vi "array -- bilinear regression 2D.vi"(7 "action":T5, 10 "fit  IN":dbl[](array[numeric])=[1.9, 2.6, 3.3, 1.0, 2.7, 3.9], 11 "xyz IN":cluster{"x":dbl[], "y":dbl[], "z":dbl[]}={"x"=[0.0, 0.0, 0.0, -1.0, -1.0, -1.0, 1.0, 1.0, 1.0], "y"=[-1.0, 0.0, 1.0, -1.0, 0.0, 1.0, -1.0, 0.0, 1.0], "z"=[1.0, 0.0, 1.0, 4.0, 1.0, 0.0, 0.0, 1.0, 4.0]}) -> (0 "output cluster":T3, 1 "fit map out":map{T4, dbl}(c390)={enum."1"=0.0, enum."x"=0.0, enum."y"=0.0, enum."xx"=1.0, enum."xy"=1.0, enum."yy"=1.0}, 2 "fit OUT":dbl[](array[numeric])=[1.0, 1.0, 1.0, 0.0, 0.0, 0.0], 3 "xyz OUT":cluster{"x":dbl[], "y":dbl[], "z":dbl[]}={"x"=[0.0, 0.0, 0.0, -1.0, -1.0, -1.0, 1.0, 1.0, 1.0], "y"=[-1.0, 0.0, 1.0, -1.0, 0.0, 1.0, -1.0, 0.0, 1.0], "z"=[1.0, 0.0, 1.0, 4.0, 1.0, 0.0, 0.0, 1.0, 4.0]})   [LabVIEW 2020]
uses:
  array -- fit control .ctl
  array -- bilinear regression 2D.ctl
  <vilib>/Analysis/Matrix/Datatypes/RealMatrix.ctl
  <vilib>/Analysis/Matrix/Datatypes/ComplexMatrix.ctl
  <vilib>/Analysis/7linalg.llb/Eigenvalue and Vectors Output Option.ctl
  <vilib>/Analysis/baseanly.llb/Matrix Type of Inverse Matrix.ctl
  <vilib>/Analysis/baseanly.llb/Real A x B.vi
  <vilib>/Analysis/Matrix/Numeric/Conversions/Array To Matrix - RA2.vi
  <vilib>/Analysis/baseanly.llb/Real Inverse Matrix.vi
  <vilib>/Analysis/Matrix/Numeric/Conversions/Matrix To Array - RM.vi
  <vilib>/Analysis/7linalg.llb/Real Eigenvalues and Vectors.vi
  <vilib>/Analysis/Matrix/Numeric/Conversions/Matrix To Array - CM.vi
  <vilib>/Analysis/NI_AALBase.lvlib
  <vilib>/Analysis/Matrix/NI_Matrix.lvlib
  <vilib>/Analysis/NI_AALPro.lvlib
panel:
  out "y OUT":dbl[](array[numeric])=[-1.0, 0.0, 1.0, -1.0, 0.0, 1.0, -1.0, 0.0, 1.0]
  out "y":dbl[](array[numeric])=[-1.0, 0.0, 1.0, -1.0, 0.0, 1.0, -1.0, 0.0, 1.0]
  out "x OUT":dbl[](array[numeric])=[0.0, 0.0, 0.0, -1.0, -1.0, -1.0, 1.0, 1.0, 1.0]
  out "z OUT":dbl[](array[numeric])=[1.0, 0.0, 1.0, 4.0, 1.0, 0.0, 0.0, 1.0, 4.0]
  out "z":dbl[](array[numeric])=[1.0, 0.0, 1.0, 4.0, 1.0, 0.0, 0.0, 1.0, 4.0]
  out "x":dbl[](array[numeric])=[0.0, 0.0, 0.0, -1.0, -1.0, -1.0, 1.0, 1.0, 1.0]
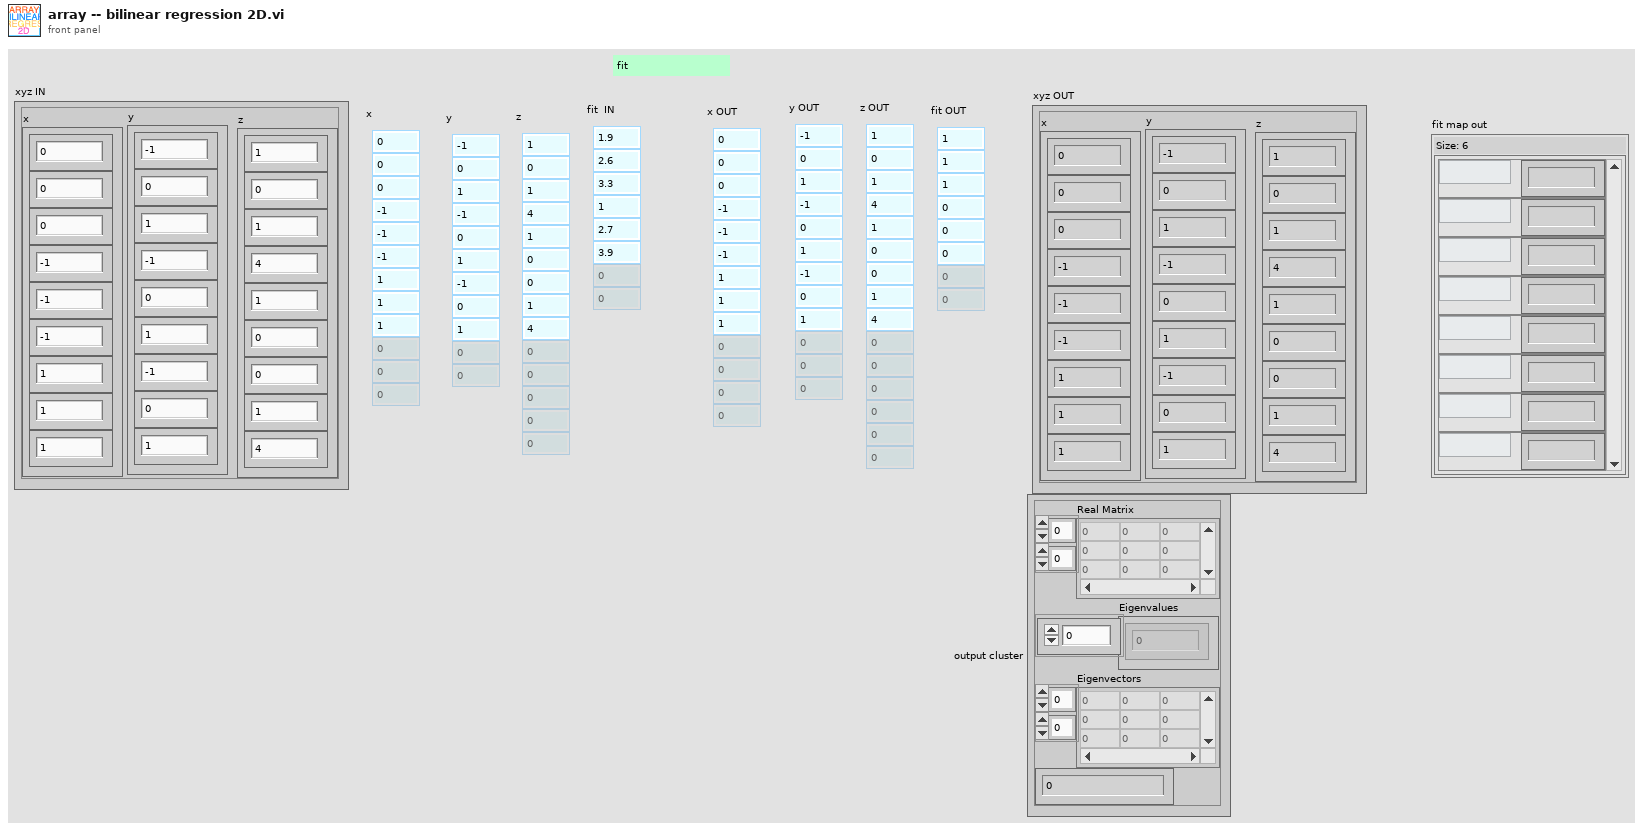
[diagram p1: front panel]
types:
  T1 = typedef "NI_Matrix.lvlib/RealMatrix.ctl" = dbl[][]
  T2 = typedef "NI_Matrix.lvlib/ComplexMatrix.ctl" = cdb[][]
  T3 = cluster{"Real Matrix":T1, "Eigenvalues":cdb[], "Eigenvectors":T2, "Numeric":cdb}
  T4 = typedef "array -- bilinear regression 2D.ctl" = enum16{"1", "x", "y", "xx", "xy", "yy", "xxy", "xyy", "yyy", "xxx", "xxyy", "xyyy", "xxxy", "yyyy", "xxxx", "xxz", "xyz", "yyz", "xz", "yz", "z"}
  T5 = typedef "array -- fit control .ctl" = enum16{"fit", "calc", "check", "init"}
  T6 = typedef "NI_AALPro.lvlib/Eigenvalue and Vectors Output Option.ctl" = i32
  T7 = typedef "NI_AALBase.lvlib/Matrix Type of Inverse Matrix.ctl" = enum32{"General", "Positive Definite", "Lower Triangular", "Upper Triangular"}
  T8 = cluster{"Real Matrix":T1, "Eigenvalues":cdb[], "Eigenvectors":T2, dbl}
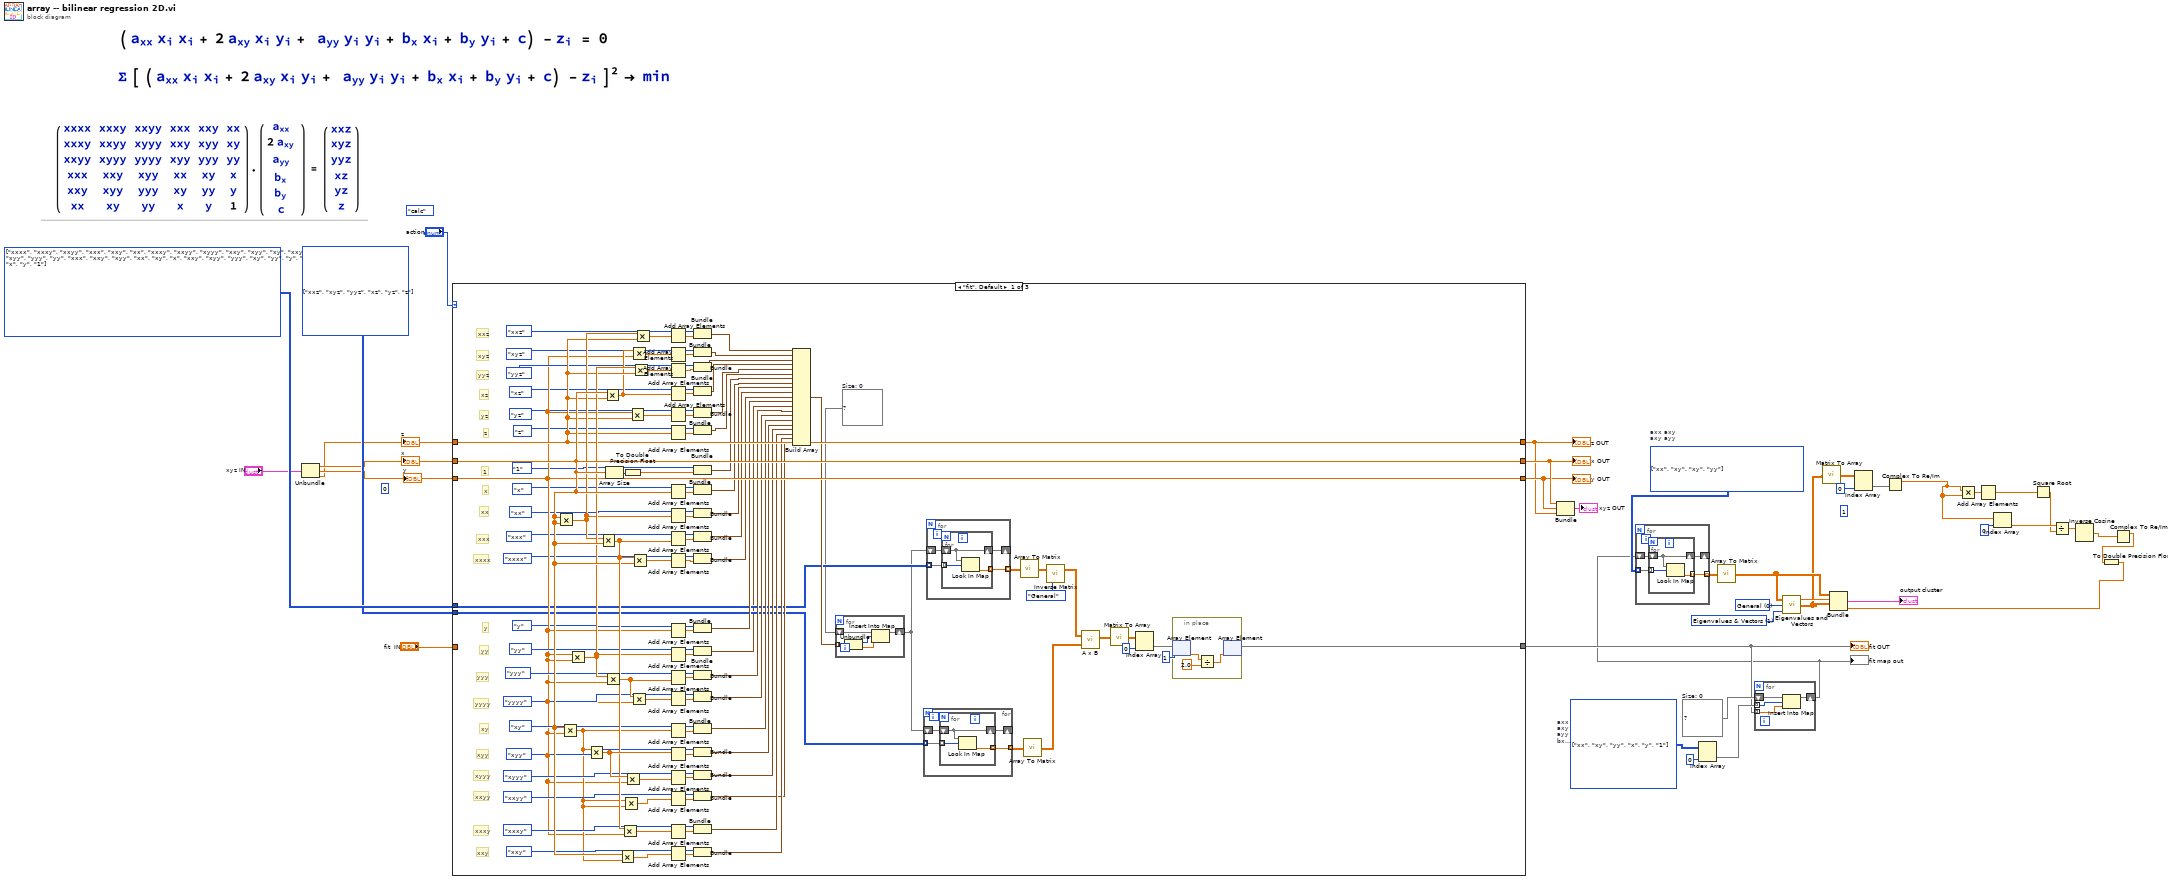
[diagram p0: block diagram]
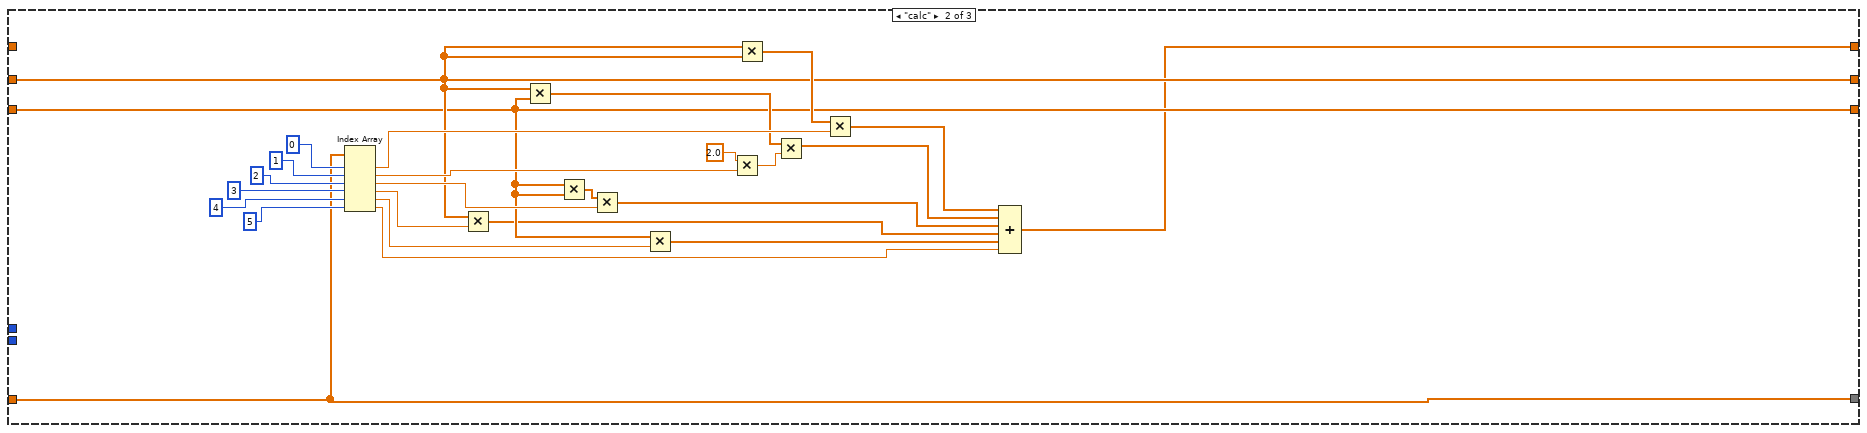
[diagram p2: hidden frame]
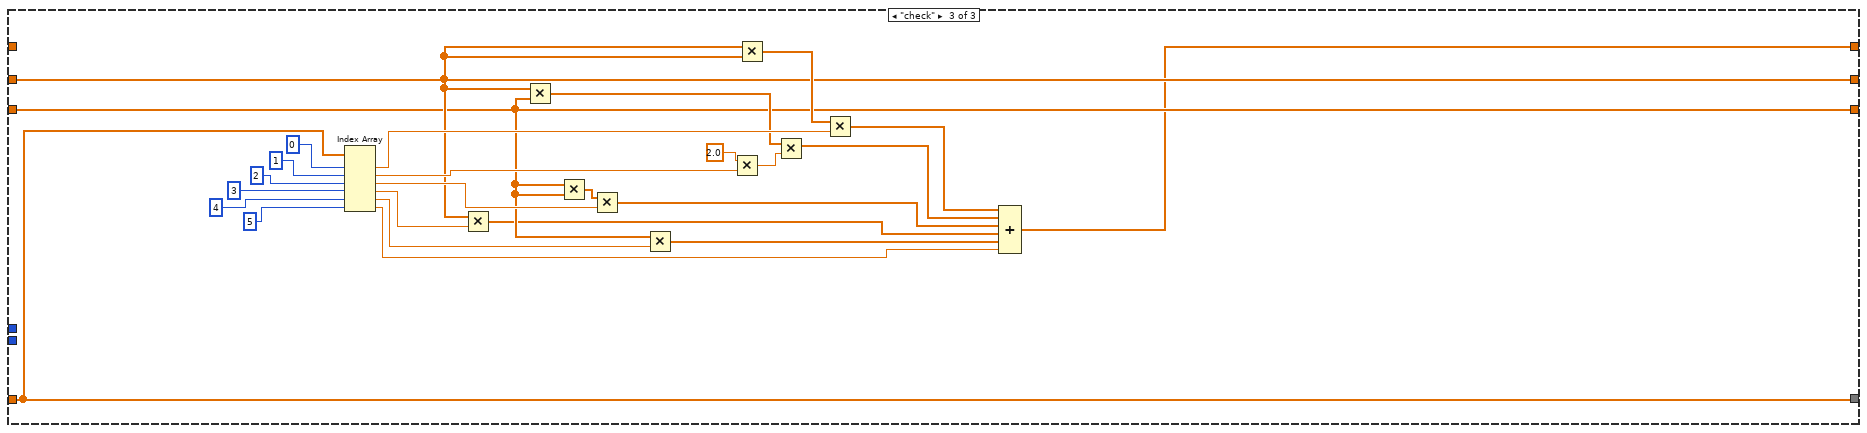
[diagram p3: hidden frame]
diagram:
  (unwired) 1 ("length")
  w18 = map{T4, dbl} {}  # Size: 0
  w20 = T4[][] [[enum."xx"], [enum."xy"], [enum."yy"], [enum."x"], [enum."y"], [enum."1"]] items=["1", "x", "y", "xx", "xy", "yy", "xxy", "xyy", "yyy", "xxx", "xxyy", "xyyy", "xxxy", "yyyy", "xxxx", "xxz", "xyz", "yyz", "xz", "yz", "z"]  # axx axy ayy bx by c
  w24 = T6 1 items=["Eigenvalues", "Eigenvalues & Vectors"] ("output option")
  w23 = 0 items=["General", "Symmetric"] ("matrix type")
  w22 = T4[][] [[enum."xx", enum."xy"], [enum."xy", enum."yy"]] items=["1", "x", "y", "xx", "xy", "yy", "xxy", "xyy", "yyy", "xxx", "xxyy", "xyyy", "xxxy", "yyyy", "xxxx", "xxz", "xyz", "yyz", "xz", "yz", "z"]  # axx axy axy ayy
  (unwired) array_--_fit_control_."calc" ("action")
  w36 = T4[][] [[enum."xxz"], [enum."xyz"], [enum."yyz"], [enum."xz"], [enum."yz"], [enum."z"]] items=["1", "x", "y", "xx", "xy", "yy", "xxy", "xyy", "yyy", "xxx", "xxyy", "xyyy", "xxxy", "yyyy", "xxxx", "xxz", "xyz", "yyz", "xz", "yz", "z"]
  w37 = T4[][] [[enum."xxxx", enum."xxxy", enum."xxyy", enum."xxx", enum."xxy", enum."xx"], [enum."xxxy", enum."xxyy", enum."xyyy", enum."xxy", enum."xyy", enum."xy"], [enum."xxyy", enum."xyyy", enum."yyyy", enum."xyy", enum."yyy", enum."yy"], [enum."xxx", enum."xxy", enum."xyy", enum."xx", enum."xy", enum."x"], [enum."xxy", enum."xyy", enum."yyy", enum."xy", enum."yy", enum."y"], [enum."xx", enum."xy", enum."yy", enum."x", enum."y", enum."1"]] items=["1", "x", "y", "xx", "xy", "yy", "xxy", "xyy", "yyy", "xxx", "xxyy", "xyyy", "xxxy", "yyyy", "xxxx", "xxz", "xyz", "yyz", "xz", "yz", "z"]
  (unwired) 0
  n1 = Unbundle("xyz IN") -> ("x"=w31:dbl[], "y"=w30:dbl[], "z"=w29:dbl[])
  "x" <- w31
  "z" <- w29
  "y" <- w30
  n2 = case shown="\"fit\", Default" "action" {
    tunnel: w29 -> [w122 _ _]
    tunnel: w31 -> [w125 w174 w200]
    tunnel: [w41 w163 w189] -> w17
    tunnel: [w122 w164 w190] -> w33
    tunnel: [w125 w174 w200] -> w35
    tunnel: "fit  IN" -> [_ w163 w189]
    tunnel: w30 -> [w94 w171 w197]
    tunnel: [w94 w171 w197] -> w34
    tunnel: w37 -> [w52 _ _]
    tunnel: w36 -> [w51 _ _]
    frame "fit", Default {
      w42 = map{T4, dbl} {}  # Size: 0
      # "z"
      # "xxz"
      # "yz"
      # "xz"
      # "yyz"
      # "xyz"
      # "xxy"
      # "xxxy"
      # "xxyy"
      # "xyyy"
      # "xyy"
      # "xy"
      # "yyyy"
      # "yyy"
      # "yy"
      # "y"
      # "1"
      # "xxxx"
      # "xxx"
      # "xx"
      # "x"
      n3 = Multiply(x=w125, y=w125) -> (x*y=w123:dbl[])
      n4 = Multiply(x=w125, y=w94) -> (x*y=w102:dbl[])
      n5 = Multiply(x=w94, y=w94) -> (x*y=w124:dbl[])
      n6 = Multiply(x=w102, y=w94) -> (x*y=w131:dbl[])
      n7 = Multiply(x=w123, y=w125) -> (x*y=w128:dbl[])
      n8 = Multiply(x=w125, y=w122) -> (x*y=w120:dbl[])
      n9 = Multiply(x=w124, y=w94) -> (x*y=w135:dbl[])
      n10 = Array Size(array=w125) -> (size(s)=w83:i32)
      n11 = Multiply(x=w125, y=w102) -> (x*y=w129:dbl[])
      n12 = Multiply(x=w128, y=w94) -> (x*y=w130:dbl[])
      n13 = Multiply(x=w102, y=w102) -> (x*y=w132:dbl[])
      n14 = To Double Precision Float(number=w83) -> (double precision float=w68:dbl)
      n15 = Multiply(x=w131, y=w94) -> (x*y=w133:dbl[])
      n16 = Multiply(x=w94, y=w122) -> (x*y=w127:dbl[])
      n17 = Multiply(x=w120, y=w94) -> (x*y=w119:dbl[])
      n18 = Multiply(x=w135, y=w94) -> (x*y=w134:dbl[])
      n19 = Multiply(x=w128, y=w125) -> (x*y=w140:dbl[])
      n20 = Multiply(x=w124, y=w122) -> (x*y=w126:dbl[])
      n21 = Multiply(x=w123, y=w122) -> (x*y=w121:dbl[])
      n22 = Add Array Elements(numeric array=w121) -> (sum=w118:dbl)
      n23 = Add Array Elements(numeric array=w119) -> (sum=w116:dbl)
      n24 = Add Array Elements(numeric array=w126) -> (sum=w113:dbl)
      n25 = Add Array Elements(numeric array=w120) -> (sum=w80:dbl)
      n26 = Add Array Elements(numeric array=w127) -> (sum=w78:dbl)
      n27 = Add Array Elements(numeric array=w122) -> (sum=w76:dbl)
      n28 = Add Array Elements(numeric array=w125) -> (sum=w85:dbl)
      n29 = Add Array Elements(numeric array=w123) -> (sum=w86:dbl)
      n30 = Add Array Elements(numeric array=w128) -> (sum=w89:dbl)
      n31 = Add Array Elements(numeric array=w140) -> (sum=w90:dbl)
      n32 = Add Array Elements(numeric array=w94) -> (sum=w93:dbl)
      n33 = Add Array Elements(numeric array=w124) -> (sum=w95:dbl)
      n34 = Add Array Elements(numeric array=w135) -> (sum=w98:dbl)
      n35 = Add Array Elements(numeric array=w134) -> (sum=w100:dbl)
      n36 = Add Array Elements(numeric array=w102) -> (sum=w59:dbl)
      n37 = Add Array Elements(numeric array=w131) -> (sum=w104:dbl)
      n38 = Add Array Elements(numeric array=w133) -> (sum=w106:dbl)
      n39 = Add Array Elements(numeric array=w132) -> (sum=w108:dbl)
      n40 = Add Array Elements(numeric array=w130) -> (sum=w110:dbl)
      n41 = Add Array Elements(numeric array=w129) -> (sum=w111:dbl)
      n42 = Bundle(array_--_bilinear_regression_2D."xxz", "Numeric"=w118) -> (w75:cluster{T4, "Numeric":dbl})  [unwired: 1 in]
      n43 = Bundle(array_--_bilinear_regression_2D."xyz", "Numeric"=w116) -> (w74:cluster{T4, "Numeric":dbl})  [unwired: 1 in]
      n44 = Bundle(array_--_bilinear_regression_2D."yyz", "Numeric"=w113) -> (w73:cluster{T4, "Numeric":dbl})  [unwired: 1 in]
      n45 = Bundle(array_--_bilinear_regression_2D."xz", "Numeric"=w80) -> (w72:cluster{T4, "Numeric":dbl})  [unwired: 1 in]
      n46 = Bundle(array_--_bilinear_regression_2D."yz", "Numeric"=w78) -> (w71:cluster{T4, "Numeric":dbl})  [unwired: 1 in]
      n47 = Bundle(array_--_bilinear_regression_2D."z", "Numeric"=w76) -> (w70:cluster{T4, "Numeric":dbl})  [unwired: 1 in]
      n48 = Bundle(array_--_bilinear_regression_2D."1", w68) -> (w69:cluster{T4, dbl})  [unwired: 1 in]
      n49 = Bundle(array_--_bilinear_regression_2D."x", "Numeric"=w85) -> (w67:cluster{T4, "Numeric":dbl})  [unwired: 1 in]
      n50 = Bundle(array_--_bilinear_regression_2D."xx", "Numeric"=w86) -> (w66:cluster{T4, "Numeric":dbl})  [unwired: 1 in]
      n51 = Bundle(array_--_bilinear_regression_2D."xxx", "Numeric"=w89) -> (w65:cluster{T4, "Numeric":dbl})  [unwired: 1 in]
      n52 = Bundle(array_--_bilinear_regression_2D."xxxx", "Numeric"=w90) -> (w64:cluster{T4, "Numeric":dbl})  [unwired: 1 in]
      n53 = Bundle(array_--_bilinear_regression_2D."y", "Numeric"=w93) -> (w63:cluster{T4, "Numeric":dbl})  [unwired: 1 in]
      n54 = Bundle(array_--_bilinear_regression_2D."yy", "Numeric"=w95) -> (w43:cluster{T4, "Numeric":dbl})  [unwired: 1 in]
      n55 = Bundle(array_--_bilinear_regression_2D."yyy", "Numeric"=w98) -> (w62:cluster{T4, "Numeric":dbl})  [unwired: 1 in]
      n56 = Bundle(array_--_bilinear_regression_2D."yyyy", "Numeric"=w100) -> (w61:cluster{T4, "Numeric":dbl})  [unwired: 1 in]
      n57 = Bundle(array_--_bilinear_regression_2D."xy", "Numeric"=w59) -> (w60:cluster{T4, "Numeric":dbl})  [unwired: 1 in]
      n58 = Bundle(array_--_bilinear_regression_2D."xyy", "Numeric"=w104) -> (w58:cluster{T4, "Numeric":dbl})  [unwired: 1 in]
      n59 = Bundle(array_--_bilinear_regression_2D."xyyy", "Numeric"=w106) -> (w57:cluster{T4, "Numeric":dbl})  [unwired: 1 in]
      n60 = Bundle(array_--_bilinear_regression_2D."xxyy", "Numeric"=w108) -> (w54:cluster{T4, "Numeric":dbl})  [unwired: 1 in]
      n61 = Bundle(array_--_bilinear_regression_2D."xxxy", "Numeric"=w110) -> (w56:cluster{T4, "Numeric":dbl})  [unwired: 1 in]
      n62 = Bundle(array_--_bilinear_regression_2D."xxy", "Numeric"=w111) -> (w55:cluster{T4, "Numeric":dbl})  [unwired: 1 in]
      n63 = Build Array(w75, w74, w73, w72, w71, w70, w69, w67, w66, w65, w64, w63, w43, w62, w61, w60, w58, w57, w56, w55, w54) -> (w53:cluster{T4, "Numeric":dbl}[])
      n64 = for {
        tunnel: w53 -> [w153] mode=indexing
        shift-right: [w154] -> w40
        shift-left: w42 -> [w155]
        n65 = Unbundle(w153) -> (w152:T4, "Numeric"=w151:dbl)
        n66 = Insert Into Map(map in=w155, key=w152, value=w151) -> (map out=w154:map{T4, dbl})  [unwired: 2 out]
      }
      n67 = for {
        shift-right: [w146] -> _
        shift-left: w40 -> [w147]
        tunnel: w51 -> [w145] mode=indexing
        tunnel: [w144] -> w48 mode=indexing
        n68 = for {
          shift-right: [w150] -> w146
          shift-left: w147 -> [w150]
          tunnel: w145 -> [w149] mode=indexing
          tunnel: [w148] -> w144 mode=indexing
          n69 = Look In Map(map=w150, key=w149) -> (value=w148:dbl)  [unwired: 1 in, 1 out]
        }
      }
      n70 = for {
        tunnel: w52 -> [w159] mode=indexing
        shift-right: [w157] -> _
        shift-left: w40 -> [w158]
        tunnel: [w156] -> w49 mode=indexing
        n71 = for {
          tunnel: w159 -> [w161] mode=indexing
          shift-right: [w162] -> w157
          shift-left: w158 -> [w162]
          tunnel: [w160] -> w156 mode=indexing
          n72 = Look In Map(map=w162, key=w161) -> (value=w160:dbl)  [unwired: 1 in, 1 out]
        }
      }
      n73 = call-poly <vilib>:"Array To Matrix.vi"("Real 2D Array"=w49) -> ("Real Matrix"=w44:T1)
      n74 = call-poly <vilib>:"Array To Matrix.vi"("Real 2D Array"=w48) -> ("Real Matrix"=w47:T1)
      n75 = call-poly <vilib>:"Inverse Matrix.vi"("matrix type"=Matrix_Type_of_Inverse_Matrix."General", "Input Matrix"=w44) -> ("Inverse Matrix"=w139:T1)  [unwired: 1 out]
      n76 = call-poly <vilib>:"A x B.vi"("B"=w47, "A"=w139) -> ("A x B"=w138:T1)  [unwired: 1 out]
      n77 = call-poly <vilib>:"Matrix To Array.vi"("Real Matrix"=w138) -> ("Real 2D Array"=w137:dbl[][])
      n78 = Index Array(array=w137, index (col)=0 ("disabled index (col)")) -> (element=w46:dbl[])  [unwired: 1 in]
      n79 = in-place {
        n80 = in-place-array #1(w46, 1) -> (w143:dbl)
        n81 = Divide(x=w143, y=2.0) -> (x/y=w141:dbl)
        n82 = in-place-array #1(w141) -> (w41:dbl[])  [unwired: 1 out]
      }
    }
    frame "calc" {
      n83 = Index Array(array=w163, index #1=0 ("index"), index #2=1 ("index"), index #3=2 ("index"), index #4=3 ("index"), index #5=4 ("index"), index #6=5 ("index")) -> (element #1=w181:dbl, element #2=w175:dbl, element #3=w177:dbl, element #4=w173:dbl, element #5=w172:dbl, element #6=w165:dbl)
      n84 = Multiply(x=w174, y=w173) -> (x*y=w167:dbl[])
      n85 = Multiply(x=w174, y=w171) -> (x*y=w180:dbl[])
      n86 = Multiply(x=w171, y=w171) -> (x*y=w178:dbl[])
      n87 = Multiply(x=w178, y=w177) -> (x*y=w168:dbl[])
      n88 = Multiply(x=w171, y=w172) -> (x*y=w166:dbl[])
      n89 = Multiply(x=2.0 ("y"), y=w175) -> (x*y=w179:dbl)
      n90 = Multiply(x=w174, y=w174) -> (x*y=w182:dbl[])
      n91 = Multiply(x=w180, y=w179) -> (x*y=w169:dbl[])
      n92 = Multiply(x=w182, y=w181) -> (x*y=w170:dbl[])
      n93 = Compound Arithmetic op=ADD(w170, w169, w168, w167, w166, w165) -> (w164:dbl[])
    }
    frame "check" {
      n94 = Index Array(array=w189, index #1=0 ("index"), index #2=1 ("index"), index #3=2 ("index"), index #4=3 ("index"), index #5=4 ("index"), index #6=5 ("index")) -> (element #1=w207:dbl, element #2=w201:dbl, element #3=w203:dbl, element #4=w199:dbl, element #5=w198:dbl, element #6=w191:dbl)
      n95 = Multiply(x=w200, y=w199) -> (x*y=w193:dbl[])
      n96 = Multiply(x=w200, y=w197) -> (x*y=w206:dbl[])
      n97 = Multiply(x=w197, y=w197) -> (x*y=w204:dbl[])
      n98 = Multiply(x=w204, y=w203) -> (x*y=w194:dbl[])
      n99 = Multiply(x=w197, y=w198) -> (x*y=w192:dbl[])
      n100 = Multiply(x=2.0 ("y"), y=w201) -> (x*y=w205:dbl)
      n101 = Multiply(x=w200, y=w200) -> (x*y=w208:dbl[])
      n102 = Multiply(x=w206, y=w205) -> (x*y=w195:dbl[])
      n103 = Multiply(x=w208, y=w207) -> (x*y=w196:dbl[])
      n104 = Compound Arithmetic op=ADD(w196, w195, w194, w193, w192, w191) -> (w190:dbl[])
    }
  }
  "fit OUT" <- w17
  "z OUT" <- w33
  "x OUT" <- w35
  "y OUT" <- w34
  n105 = Bundle("x"=w35, "y"=w34, "z"=w33) -> (→"xyz OUT":cluster{"x":dbl[], "y":dbl[], "z":dbl[]})  [unwired: 1 in]
  n106 = Index Array(array=w20, index (col)=0 ("disabled index (col)")) -> (element=w21:T4[])  [unwired: 1 in]
  n107 = for {
    shift-right: [w217] -> w16
    shift-left: w18 -> [w218]
    tunnel: w21 -> [w216] mode=indexing
    tunnel: w17 -> [w215] mode=indexing
    n108 = Insert Into Map(map in=w218, key=w216, value=w215) -> (map out=w217:map{T4, dbl})  [unwired: 2 out]
  }
  "fit map out" <- w16
  n109 = for {
    tunnel: w22 -> [w222] mode=indexing
    shift-right: [w220] -> _
    shift-left: w16 -> [w221]
    tunnel: [w219] -> w25 mode=indexing
    n110 = for {
      tunnel: w222 -> [w224] mode=indexing
      shift-right: [w225] -> w220
      shift-left: w221 -> [w225]
      tunnel: [w223] -> w219 mode=indexing
      n111 = Look In Map(map=w225, key=w224) -> (value=w223:dbl)  [unwired: 1 in, 1 out]
    }
  }
  n112 = call-poly <vilib>:"Array To Matrix.vi"("Real 2D Array"=w25) -> ("Real Matrix"=w26:T1)
  n113 = call-poly <vilib>:"Eigenvalues and Vectors.vi"("output option"=w24, "matrix type"=w23, "Input Matrix"=w26) -> ("Eigenvectors"=w9:T2, "Eigenvalues"=w27:cdb[])  [unwired: 1 out]
  n114 = call-poly <vilib>:"Matrix To Array.vi"("Complex Matrix"=w9) -> ("Complex 2D Array"=w8:cdb[][])
  n115 = Index Array(array=w8, index (col)=0 ("disabled index (col)")) -> (element=w6:cdb[])  [unwired: 1 in]
  n116 = Complex To Re/Im(x + iy=w6) -> (x=w5:dbl[])  [unwired: 1 out]
  n117 = Multiply(x=w5, y=w5) -> (x*y=w14:dbl[])
  n118 = Add Array Elements(numeric array=w14) -> (sum=w7:dbl)
  n119 = Index Array(array=w5, index=0 ("disabled index (col)")) -> (element=w12:dbl)
  n120 = Square Root(x=w7) -> (sqrt(x)=w11:dbl)
  n121 = Divide(x=w12, y=w11) -> (x/y=w10:dbl)
  n122 = Inverse Cosine(1:w10) -> (0:w2:dbl)
  n123 = Complex To Re/Im(x + iy=w2) -> (x=w1:dbl)  [unwired: 1 out]
  n124 = To Double Precision Float(number=w1) -> (double precision float=w4:dbl)
  n125 = Bundle("Real Matrix"=w26, "Eigenvalues"=w27, "Eigenvectors"=w9, w4) -> (→"output cluster":T8)  [unwired: 1 in]
